vi "GoTo PID mirante.vi"(9 "Aim":dbl[](array[numeric]), 10 "Target":dbl[](array[numeric]), 11 "Position":dbl[](array[numeric])) -> (3 "Velocity":dbl[](array[numeric]))   [LabVIEW 2016]
uses:
  <vilib>/Analysis/coordinate.llb/2D Cartesian Coordinate Rotation (Scalar).vi
  <vilib>/addons/control/pid/pid.llb/PID (DBL Array).vi
  <vilib>/addons/control/pid/pid.llb/PID (DBL).vi
  <vilib>/addons/control/pid/NI_PID_pid.lvlib
  <vilib>/Analysis/NI_AALPro.lvlib
panel:
  in  "Constantes theta":T1={"proportional gain (Kc)"=1.0, "integral time (Ti, min)"=0.0, "derivative time (Td, min)"=0.0}
  in  "Constantes Vel":T2(array[cluster])=[{"proportional gain (Kc)"=0.05, "integral time (Ti, min)"=0.0, "derivative time (Td, min)"=0.0}, {"proportional gain (Kc)"=0.05, "integral time (Ti, min)"=0.0, "derivative time (Td, min)"=0.0}]
  out "Waveform Chart":dbl(graph)
  out "Numeric":dbl
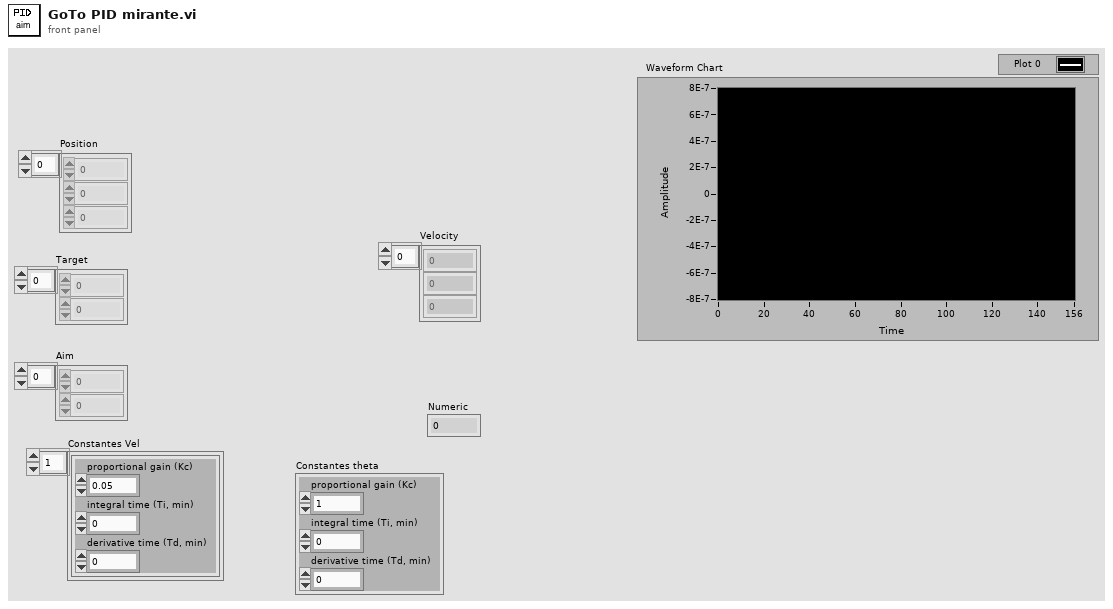
[diagram p1: front panel]
types:
  T1 = cluster{"proportional gain (Kc)":dbl, "integral time (Ti, min)":dbl, "derivative time (Td, min)":dbl}
  T2 = cluster{"proportional gain (Kc)":dbl, "integral time (Ti, min)":dbl, "derivative time (Td, min)":dbl}[]
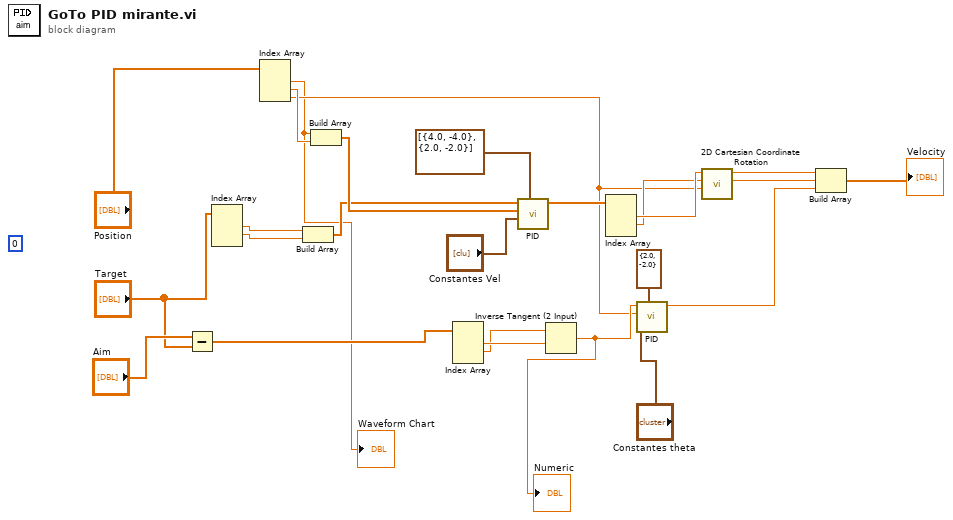
[diagram p0: block diagram]
diagram:
  (unwired) 0 ("index")
  n1 = Subtract(x="Aim", y="Target") -> (x-y=w18:dbl[])
  n2 = Index Array(array="Target") -> (element #1=w6:dbl, element #2=w5:dbl)  [unwired: 3 in, 1 out]
  n3 = Index Array(array="Position") -> (element #1=w1:dbl, element #2=w3:dbl, element #3=w2:dbl)  [unwired: 3 in]
  "Waveform Chart" <- w1
  n4 = Build Array(w6, w5) -> (w4:dbl[])
  n5 = Build Array(w1, w3) -> (w8:dbl[])
  n6 = Index Array(array=w18) -> (element #1=w17:dbl, element #2=w16:dbl)  [unwired: 3 in, 1 out]
  n7 = call-poly <vilib>:"PID.vi"("output range"=cluster{"output high":dbl, "output low":dbl}[] [{"output high"=4.0, "output low"=-4.0}, {"output high"=2.0, "output low"=-2.0}], "PID gains"="Constantes Vel", "process variable"=w8, "setpoint"=w4) -> ("output"=w22:dbl[])  [unwired: 6 in, 1 out]
  n8 = Inverse Tangent (2 Input)(1:w17, 2:w16) -> (0:w9:dbl)
  "Numeric" <- w9
  n9 = Index Array(array=w22) -> (element #1=w21:dbl, element #2=w20:dbl)  [unwired: 3 in, 1 out]
  n10 = call-poly <vilib>:"PID.vi"("output range"=cluster{"output high":dbl, "output low":dbl} {"output high"=2.0, "output low"=-2.0}, "PID gains"="Constantes theta", "process variable"=w2, "setpoint"=w9) -> ("output"=w13:dbl)  [unwired: 6 in, 1 out]
  n11 = call-poly <vilib>:"2D Cartesian Coordinate Rotation.vi"("theta"=w2, "y"=w20, "x"=w21) -> ("y out"=w14:dbl, "x out"=w15:dbl)  [unwired: 6 in, 1 out]
  n12 = Build Array(w15, w14, w13) -> (→"Velocity":dbl[])
